vi "Join_arrays.vi"(8 "Array to be added":dbl[][](array[numeric]), 11 "Old Array":dbl[][](array[numeric])) -> (3 "Output array":dbl[][](array[numeric]))   [LabVIEW 2021]
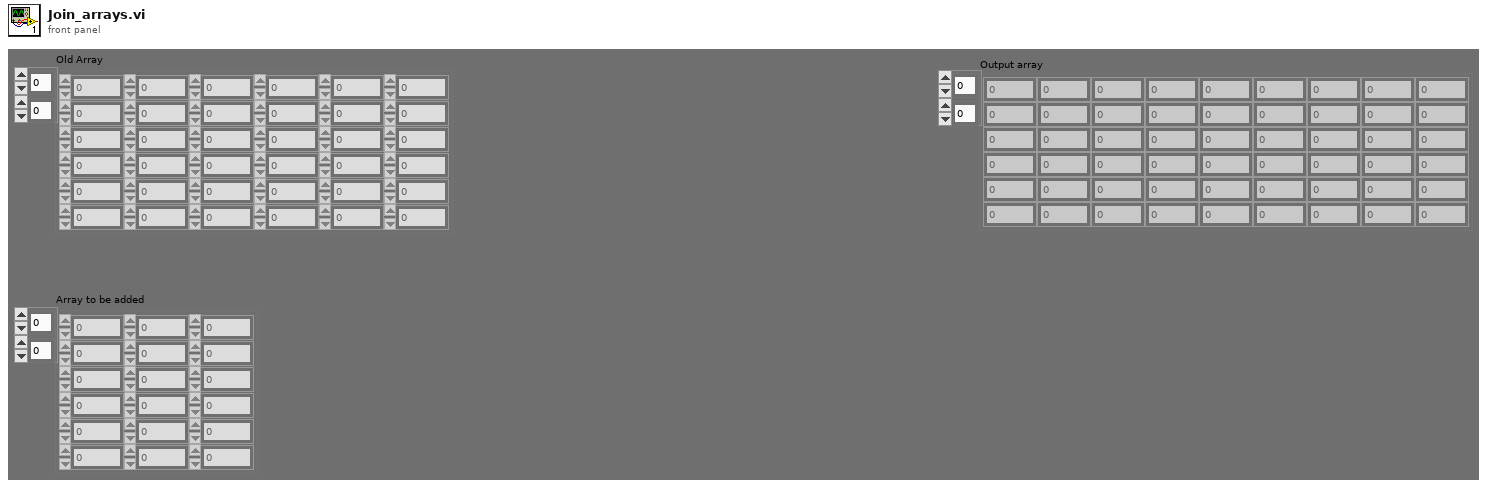
[diagram p1: front panel]
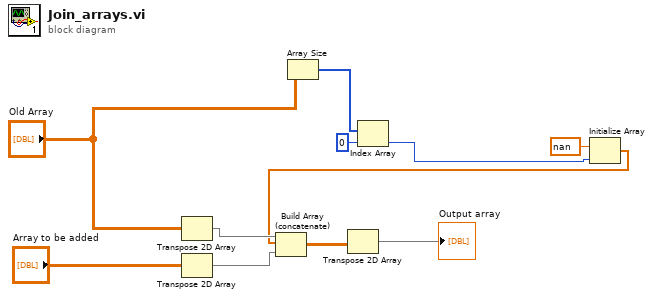
[diagram p0: block diagram]
diagram:
  n1 = Transpose 2D Array(2D array="Old Array") -> (transposed array=w10:dbl[][])
  n2 = Transpose 2D Array(2D array="Array to be added") -> (transposed array=w2:dbl[][])
  n3 = Array Size(array="Old Array") -> (size(s)=w7:i32[])
  n4 = Index Array(array=w7, index=0) -> (element=w3:i32)
  n5 = Initialize Array(nan ("element"), w3) -> (w1:dbl[])
  n6 = Build Array (concatenate)(w10, w1, w2) -> (w9:dbl[][])
  n7 = Transpose 2D Array(2D array=w9) -> (transposed array=→"Output array":dbl[][])
